vi "Connect_to_BSA_IP.vi"() -> (0 "error out":errorcluster, 1 "BSA":refnum<k7>)   [LabVIEW 2010]
uses:
  Globals/LDA_meas_global_1.vi
panel:
  in  "BSACtrl.IBSA":refnum<k7>
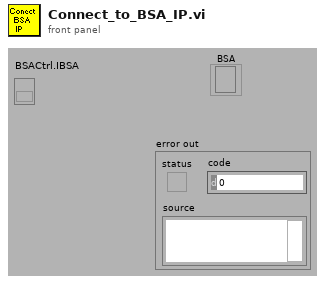
[diagram p1: front panel]
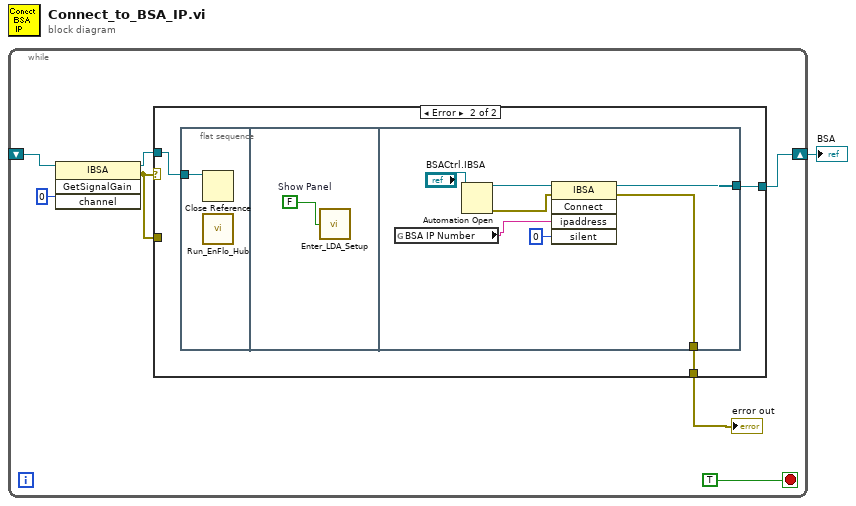
[diagram p0: block diagram]
diagram:
  n1 = while {
    shift-right: [w6] -> w1
    shift-left: _ -> [w7]
    stop <- TRUE stop-if-true
    n2 = invoke class="IBSA" method="GetSignalGain"(reference=w7, "channel"=0) -> (reference out=w5:refnum<k7>, error out=w2:errorcluster)  [unwired: 2 in, 2 out]
    n3 = case shown="Error" w2 {
      tunnel: [w10 w13] -> w6
      tunnel: w5 -> [w10 w11]
      tunnel: [w9 w12] -> w3
      tunnel: w2 -> [w9 _]
      frame No Error {
      }
      frame Error {
        n4 = flat-sequence {
          tunnel: w11 -> [w14]
          tunnel: [w17] -> w13
          tunnel: [w16] -> w12
          frame #0 {
            n5 = Close Reference(reference=w14) -> ()  [unwired: 1 in, 1 out]
            n6 = call "Run_EnFlo_Hub.vi"() -> ()  [unwired: 8 out]
          }
          frame #1 {
            w15 = FALSE  # Show Panel
            n7 = call "Enter_LDA_Setup.vi"("Show Panel"=w15) -> ()
          }
          frame #2 {
            n8 = global read "LDA_meas_global_1.vi" "BSA IP Number"() -> (w18:string)
            n9 = Automation Open(Automation Refnum="BSACtrl.IBSA") -> (Automation Refnum=w21:refnum<k7>, error out=w20:errorcluster)  [unwired: 2 in, 1 out]
            n10 = invoke class="IBSA" method="Connect"(reference=w21, error in=w20, "ipaddress"=w18, "silent"=0) -> (reference out=w17:refnum<k7>, error out=w16:errorcluster)  [unwired: 1 in, 3 out]
          }
        }
      }
    }
    "error out" <- w3
  }
  "BSA" <- w1
